vi "LinearFilter_Calculate.vi"(9 "Input":dbl format="%13.5p", 11 "In LINEAR_FILTER":T1 {"Outputs" format="%13.5p"; "Inputs" format="%13.5p"; "OutputGains" format="%13.5p"; "InputGains" format="%13.5p"}) -> (1 "Output":dbl format="%13.5p", 3 "Out LINEAR_FILTER":T1 {"Outputs" format="%13.5p"; "Inputs" format="%13.5p"; "OutputGains" format="%13.5p"; "InputGains" format="%13.5p"})   [LabVIEW 2019, in "Trajectory_Library.lvlib"]
doc: "Calculates the next value of the filter. To work correctly this must be called periodically\n\nInputs:\n - inLinearfilter - Linear filter data structure\n - input - Current input value.\n \nOutputs:\n - outLinearfilter - Updated linear filter data structurea\n - output - The filtered value at this step"
uses:
  Trajectory_Library.lvlib
  LINEAR_FILTER.ctl
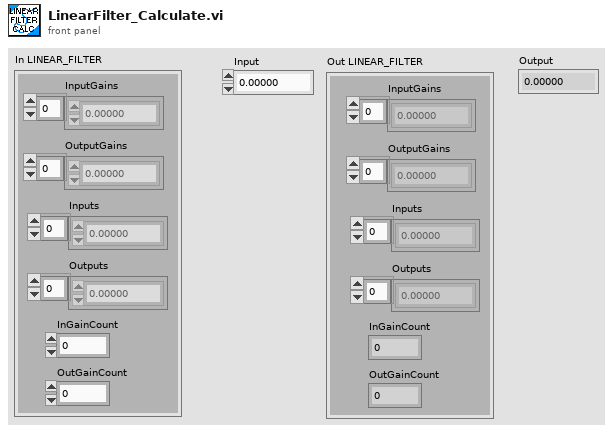
[diagram p1: front panel]
types:
  T1 = typedef "Trajectory_Library.lvlib/LINEAR_FILTER.ctl" = cluster{"InputGains":dbl[], "OutputGains":dbl[], "Inputs":dbl[], "Outputs":dbl[], "InGainCount":i32, "OutGainCount":i32}
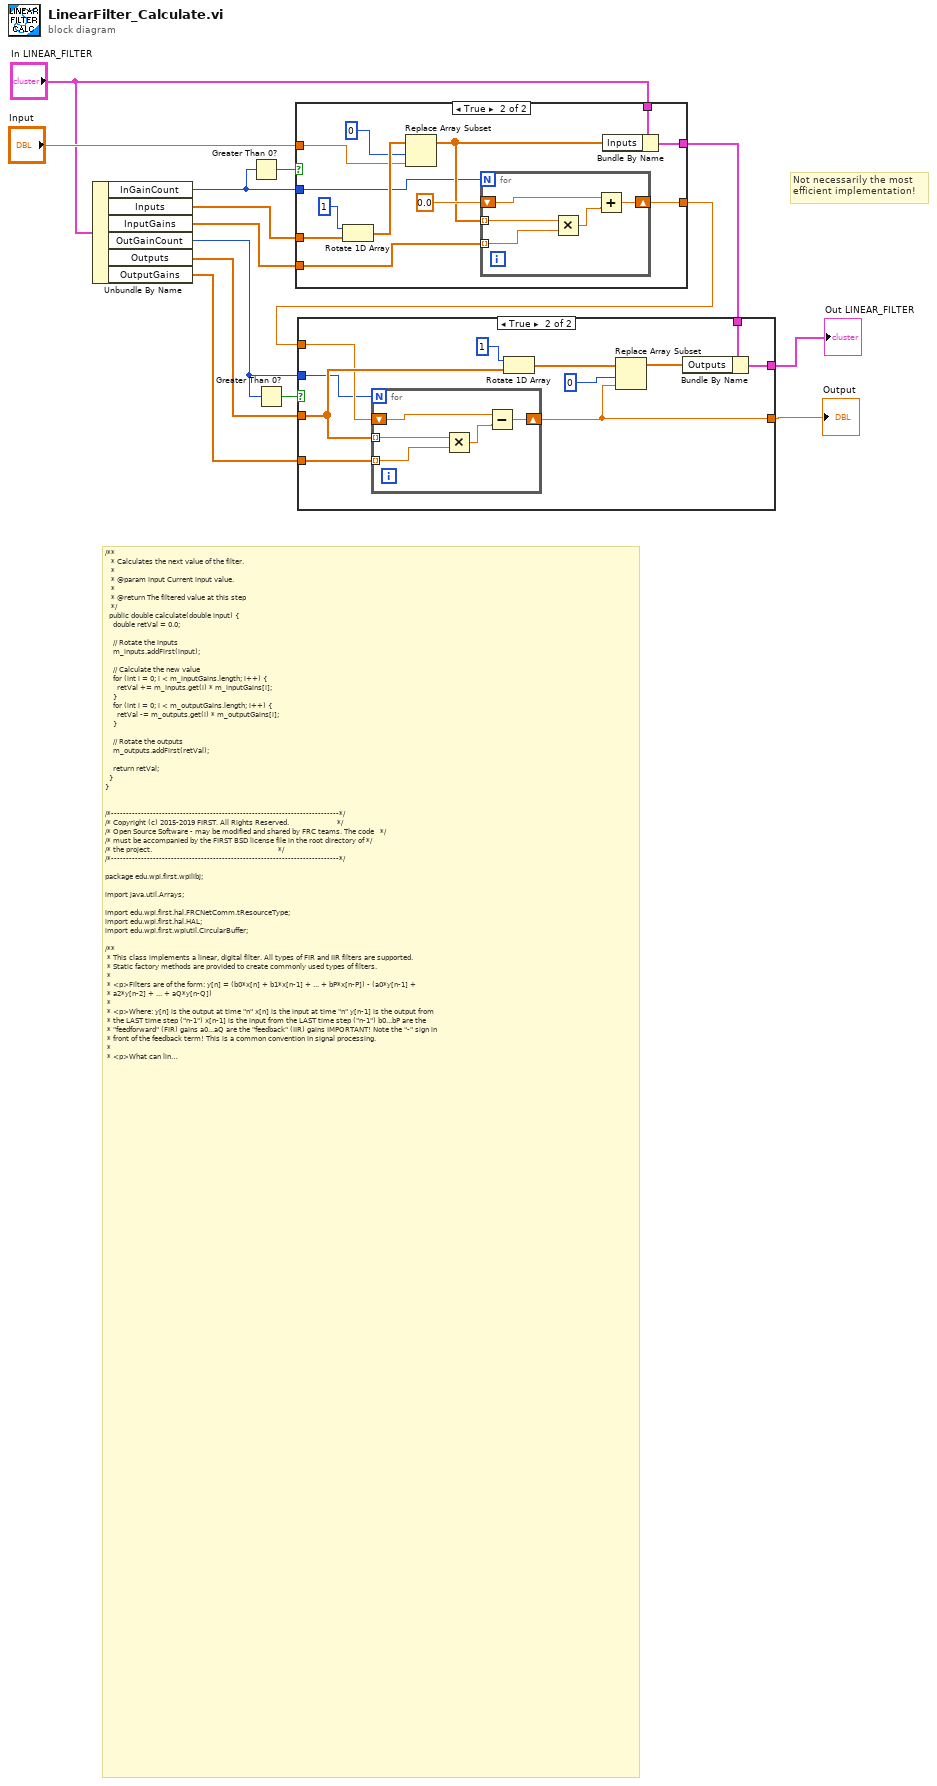
[diagram p0: block diagram]
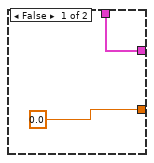
[diagram p3: hidden frame]
diagram:
  # "Not necessarily the most\nefficient implementation!"
  # "/**\n   * Calculates the next value of the filter.\n   *\n   * @param input Current input value.\n   *\n   * @return The filtered value at this step\n   */\n  public double calculate(double input) {\n    double retVal = 0.0;\n\n    // Rotate the inputs\n    m_inputs.addFirst(input);\n\n    // Calculate the new value\n    for (int i = 0; i < m_inputGains.length; i++) {\n      retVal += m_inputs.get(i) * m_inputGains[i];\n    }\n    for (int i = 0; i < m_outputGains.length; i++) {\n      retVal -= m_outputs.get(i) * m_outputGains[i];\n    }\n\n    // Rotate the outputs\n    m_outputs.addFirst(retVal);\n\n    return retVal;\n  }\n}\n\n\n/*----------------------------------------------------------------------------*/\n/* Copyright (c) 2015-2019 FIRST. All Rights Reserved.                        */\n/* Open Source Software - may be modified and shared by FRC teams. The code   */\n/* must be accompanied by the FIRST BSD license file in the root directory of */\n/* the project.                                                               */\n/*----------------------------------------------------------------------------*/\n\npackage edu.wpi.first.wpilibj;\n\nimport java.util.Arrays;\n\nimport edu.wpi.first.hal.FRCNetComm.tResourceType;\nimport edu.wpi.first.hal.HAL;\nimport edu.wpi.first.wpiutil.CircularBuffer;\n\n/**\n * This class implements a linear, digital filter. All types of FIR and IIR filters are supported.\n * Static factory methods are provided to create commonly used types of filters.\n *\n * <p>Filters are of the form: y[n] = (b0*x[n] + b1*x[n-1] + ... + bP*x[n-P]) - (a0*y[n-1] +\n * a2*y[n-2] + ... + aQ*y[n-Q])\n *\n * <p>Where: y[n] is the output at time \"n\" x[n] is the input at time \"n\" y[n-1] is the output from\n * the LAST time step (\"n-1\") x[n-1] is the input from the LAST time step (\"n-1\") b0...bP are the\n * \"feedforward\" (FIR) gains a0...aQ are the \"feedback\" (IIR) gains IMPORTANT! Note the \"-\" sign in\n * front of the feedback term! This is a common convention in signal processing.\n *\n * <p>What can linear filters do? Basically, they can filter, or diminish, the effects of\n * undesirable input frequencies. High frequencies, or rapid changes, can be indicative of sensor\n * noise or be otherwise undesirable. A \"low pass\" filter smooths out the signal, reducing the\n * impact of these high frequency components.  Likewise, a \"high pass\" filter gets rid of\n * slow-moving signal components, letting you detect large changes more easily.\n *\n * <p>Example FRC applications of filters: - Getting rid of noise from an analog sensor input (note:\n * the roboRIO's FPGA can do this faster in hardware) - Smoothing out joystick input to prevent the\n * wheels from slipping or the robot from tipping - Smoothing motor commands so that unnecessary\n * strain isn't put on electrical or mechanical components - If you use clever gains, you can make a\n * PID controller out of this class!\n *\n * <p>For more on filters, we highly recommend the following articles:<br>\n * https://en.wikipedia.org/wiki/Linear_filter<br>\n * https://en.wikipedia.org/wiki/Iir_filter<br>\n * https://en.wikipedia.org/wiki/Fir_filter<br>\n *\n * <p>Note 1: calculate() should be called by the user on a known, regular period. You can use a\n * Notifier for this or do it \"inline\" with code in a periodic function.\n *\n * <p>Note 2: For ALL filters, gains are necessarily a function of frequency. If you make a filter\n * that works well for you at, say, 100Hz, you will most definitely need to adjust the gains if you\n * then want to run it at 200Hz! Combining this with Note 1 - the impetus is on YOU as a developer\n * to make sure calculate() gets called at the desired, constant frequency!\n */"
  n1 = Unbundle By Name("In LINEAR_FILTER") -> ("InGainCount"=w2:i32, "Inputs"=w12:dbl[], "InputGains"=w9:dbl[], "OutGainCount"=w1:i32, "Outputs"=w11:dbl[], "OutputGains"=w8:dbl[])
  n2 = Greater Than 0?(x=w2) -> (x > 0?=w14:bool)
  n3 = Greater Than 0?(x=w1) -> (x > 0?=w13:bool)
  n4 = case shown="True" w14 {
    tunnel: w12 -> [_ w26]
    tunnel: "Input" -> [_ w23]
    tunnel: w9 -> [_ w18]
    tunnel: "In LINEAR_FILTER" -> [w16 w28]
    tunnel: [w16 w27] -> w6
    tunnel: [0.0 w20] -> w4
    tunnel: w2 -> [_ w17]
    frame False {
    }
    frame True {
      n5 = Rotate 1D Array(1:w26, 2:1 ("n")) -> (0:w24:dbl[])
      n6 = Replace Array Subset(array=w24, new element=w23, index=0) -> (w19:dbl[])
      n7 = for {
        N: w17 -> [_]
        shift-right: [w33] -> w20
        shift-left: 0.0 -> [w32]
        tunnel: w19 -> [w30] mode=indexing
        tunnel: w18 -> [w29] mode=indexing
        n8 = Multiply(x=w30, y=w29) -> (x*y=w31:dbl)
        n9 = Add(x=w32, y=w31) -> (x+y=w33:dbl)
      }
      n10 = Bundle By Name(cluster=w28, "Inputs"=w19) -> (w27:T1)
    }
  }
  n11 = case shown="True" w13 {
    tunnel: w11 -> [_ w39]
    tunnel: w8 -> [_ w38]
    tunnel: w6 -> [w35 w46]
    tunnel: [w35 w45] -> w5
    tunnel: w4 -> [w34 w37]
    tunnel: [w34 w40] -> w3
    tunnel: w1 -> [_ w36]
    frame False {
    }
    frame True {
      n12 = for {
        N: w36 -> [_]
        shift-right: [w51] -> w40
        shift-left: w37 -> [w50]
        tunnel: w39 -> [w48] mode=indexing
        tunnel: w38 -> [w47] mode=indexing
        n13 = Multiply(x=w48, y=w47) -> (x*y=w49:dbl)
        n14 = Subtract(x=w50, y=w49) -> (x-y=w51:dbl)
      }
      n15 = Rotate 1D Array(1:w39, 2:1 ("n")) -> (0:w43:dbl[])
      n16 = Replace Array Subset(array=w43, new element=w40, index=0) -> (w41:dbl[])
      n17 = Bundle By Name(cluster=w46, "Outputs"=w41) -> (w45:T1)
    }
  }
  "Out LINEAR_FILTER" <- w5
  "Output" <- w3
